vi "Get cif_management_common_MonitorU64.vi"(8 "error in (no error)":errorcluster, 11 "gRPCid":T1) -> (0 "error out":errorcluster, 2 "package_templatemessage":T2, 3 "gRPCid out":T1)   [LabVIEW 2021, in "CIF_PluginLoader_server.lvlib"]
uses:
  CIF_PluginLoader_server.lvlib
  cif_management_common_MonitorU64.ctl
  <vilib>/gRPC/LabVIEW gRPC Library/Shared/grpcId.ctl
  cif_management_common_MonitorU64_Flat.ctl
  2ed25e12-861d-4677-8ead-ace2906b2041.vi
  <vilib>/gRPC/LabVIEW gRPC Library/Shared/TranslateGrpcError.vi
  <vilib>/gRPC/LabVIEW gRPC Library/Server API/Server/Get Server DLL Path.vi
  <vilib>/Utility/error.llb/Error Cluster From Error Code.vi
  <vilib>/gRPC/LabVIEW gRPC Library/grpc-lvsupport-release.lvlib
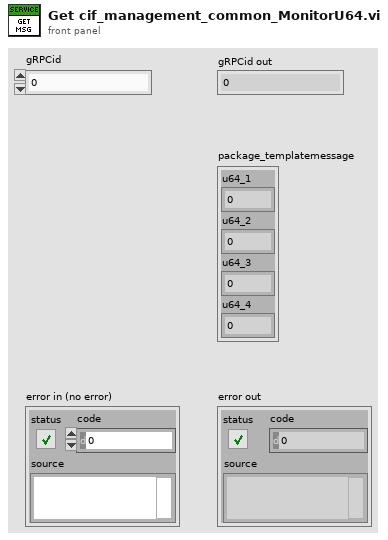
[diagram p1: front panel]
types:
  T1 = typedef "grpc-lvsupport-release.lvlib/grpcId.ctl" = u64
  T2 = typedef "CIF_PluginLoader_server.lvlib/cif_management_common_MonitorU64.ctl" = cluster{"u64_1":u64, "u64_2":u64, "u64_3":u64, "u64_4":u64}
  T3 = typedef "CIF_PluginLoader_server.lvlib/cif_management_common_MonitorU64_Flat.ctl" = cluster{"u64_1":u64, "u64_2":u64, "u64_3":u64, "u64_4":u64}
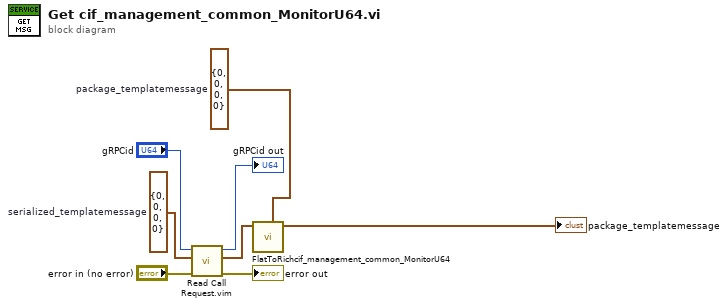
[diagram p0: block diagram]
diagram:
  w6 = T3 {"u64_1"=0, "u64_2"=0, "u64_3"=0, "u64_4"=0}  # serialized_templatemessage
  w5 = T2 {"u64_1"=0, "u64_2"=0, "u64_3"=0, "u64_4"=0}  # package_templatemessage
  n1 = call "Read Call Request.vim"("error in"="error in (no error)", "Request Type"=w6, "gRPCid in"="gRPCid") -> ("error out"=→"error out":errorcluster, "Request Data"=w4:T3, "gRPCid out"=→"gRPCid out":T1)  [unwired: 6 in]
  n2 = call "FlatToRichcif_management_common_MonitorU64.vi"("OutputClusterType"=w5, "InputCluster"=w4) -> ("OutputCluster"=→"package_templatemessage":T2)  [unwired: 9 in]
